vi "attack.vi"   [LabVIEW 2017]
uses:
  GlobalVar.vi
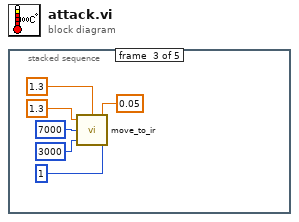
[diagram p0: block diagram]
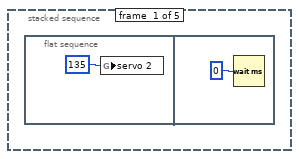
[diagram p2: hidden frame]
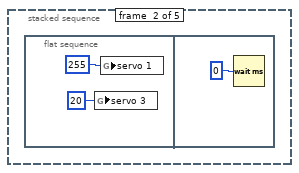
[diagram p3: hidden frame]
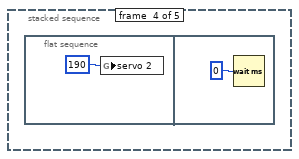
[diagram p4: hidden frame]
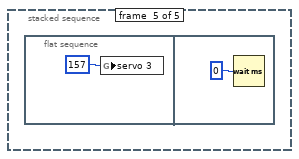
[diagram p5: hidden frame]
diagram:
  n1 = stacked-sequence {
    frame #0 {
      n2 = flat-sequence {
        frame #0 {
          n3 = global write "GlobalVar.vi" "servo 2"(u8 135 ("servo 1")) -> ()
        }
        frame #1 {
          n4 = Wait (ms)(milliseconds to wait=u32 0) -> ()  [unwired: 1 out]
        }
      }
    }
    frame #1 {
      n5 = flat-sequence {
        frame #0 {
          n6 = global write "GlobalVar.vi" "servo 3"(u8 20 ("servo 3")) -> ()
          n7 = global write "GlobalVar.vi" "servo 1"(u8 255 ("servo 1")) -> ()
        }
        frame #1 {
          n8 = Wait (ms)(milliseconds to wait=u32 0) -> ()  [unwired: 1 out]
        }
      }
    }
    frame #2 {
      n9 = call "move_to_ir.vi"("step"=1, "precision"=0.05, "target_ir_r"=1.3 ("target_ir_l"), "samples"=3000, "delay_after"=u32 7000, "target_ir_l"=1.3) -> ()
    }
    frame #3 {
      n10 = flat-sequence {
        frame #0 {
          n11 = global write "GlobalVar.vi" "servo 2"(u8 190 ("servo 1")) -> ()
        }
        frame #1 {
          n12 = Wait (ms)(milliseconds to wait=u32 0) -> ()  [unwired: 1 out]
        }
      }
    }
    frame #4 {
      n13 = flat-sequence {
        frame #0 {
          n14 = global write "GlobalVar.vi" "servo 3"(u8 157 ("servo 1")) -> ()
        }
        frame #1 {
          n15 = Wait (ms)(milliseconds to wait=u32 0) -> ()  [unwired: 1 out]
        }
      }
    }
  }
